vi "CI Server Build Package.vi"() -> ()   [LabVIEW 2016]
doc: "This VI is an example of a VI that can build a VIPM Package when the Build button is pushed or when called from the command line."
uses:
  <vilib>/SourceControl/sccapi/SCCAPI Refnum.ctl
  <userlib>/_OpenG.lib/file/file.llb/File Exists - Scalar__ogtk.vi
  <userlib>/_OpenG.lib/file/file.llb/Valid Path - Traditional__ogtk.vi
  <vilib>/AppBuilder/AB_API_Simple/Build (path).vi
  <vilib>/AppBuilder/AB_API_Simple/NI_App_Builder_API.lvlib
  LabVIEW Project API__icon_lib_labview_project_api Folder/LabVIEW Project API__icon_lib_labview_project_api.lvlib
  <vilib>/SourceControl/sccapi/NI_SCC.lvlib
panel:
  out "Build Number":u32
  out "Tests Pass":bool
  out "Unit Test Results":string
  in  "VI Package Build Spec path":path
  in  "button_build":bool
  out "Progress status":string
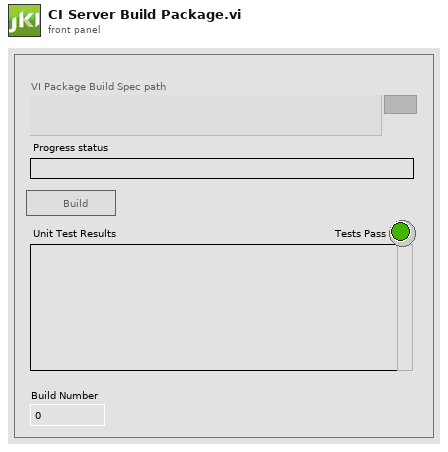
[diagram p1: front panel]
types:
  T1 = enum32{"invalid app kind", "Development System", "Run Time System", "Student Edition", "Embedded LabVIEW", "Evaluation", "Custom"}
  T2 = enum8{"Enabled", "Disabled", "Disabled and Grayed Out"}
  T3 = enum32{"Invalid", "Standard", "Closed", "Hidden", "Minimized", "Maximized"}
  T4 = typedef "NI_SCC.lvlib/SCCAPI Refnum.ctl" = refnum<k1>
  T5 = cluster{"Core":cluster{"Current VI Reference":refnum<vi>, "Close Panel on Exit?":bool}, "Paths":cluster{"Package Spec file path":path, "Unit Test Path":path}, "Building":bool, "RunningAsCmdLine":bool, "SCC Ref":T4, "Proj Ref":refnum<vi>, "Proj Item":refnum<vi>, "CmdLineArgs":cluster{"BuildNumber":u32, "Error Path":path, "Running Path":path, "Settings Path":path}}
  T6 = cluster{"BuildNumber":u32, "Error Path":path, "Running Path":path, "Settings Path":path}
  T7 = cluster{"Package Spec file path":path, "Unit Test Path":path}
  T8 = cluster{"Current VI Reference":refnum<vi>, "Close Panel on Exit?":bool}
  T9 = cluster{"Major":u16, "Minor":u16, "Fix":u16, "Build":u16}
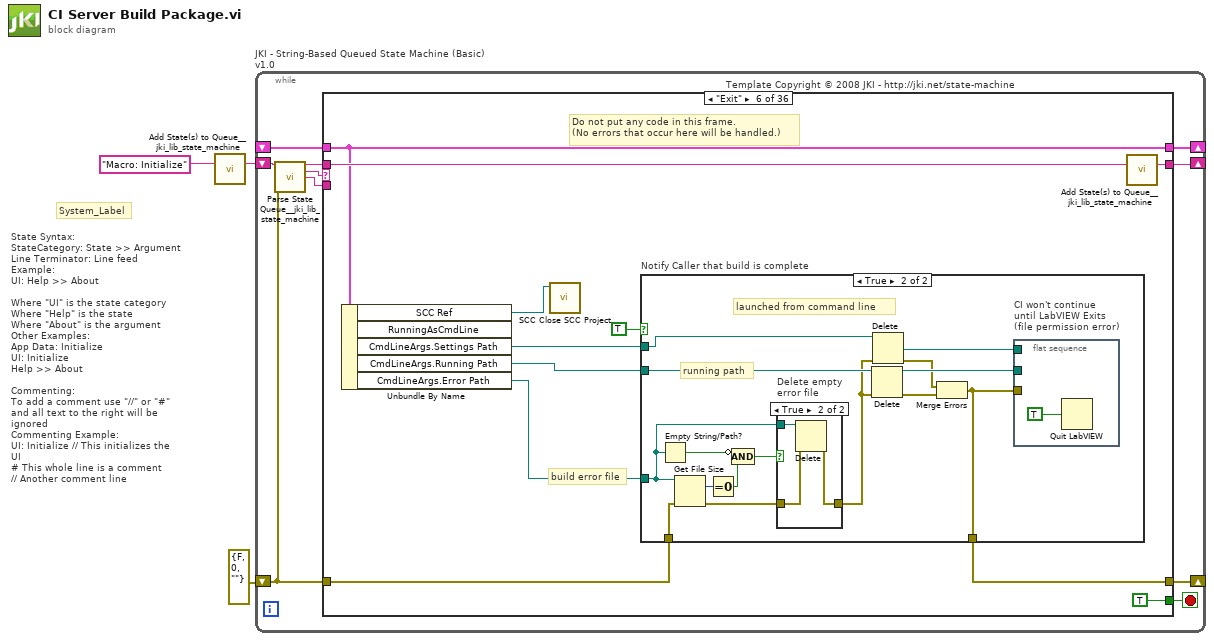
[diagram p0: block diagram]
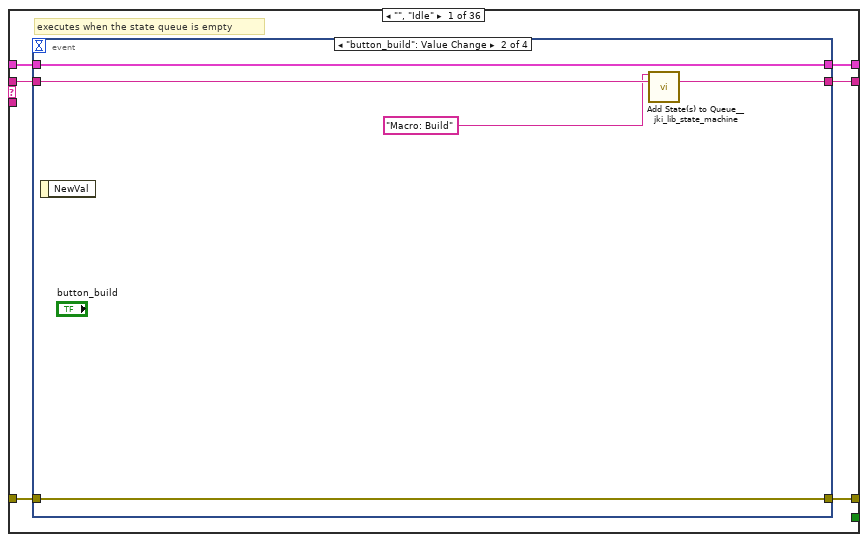
[diagram p2: hidden frame]
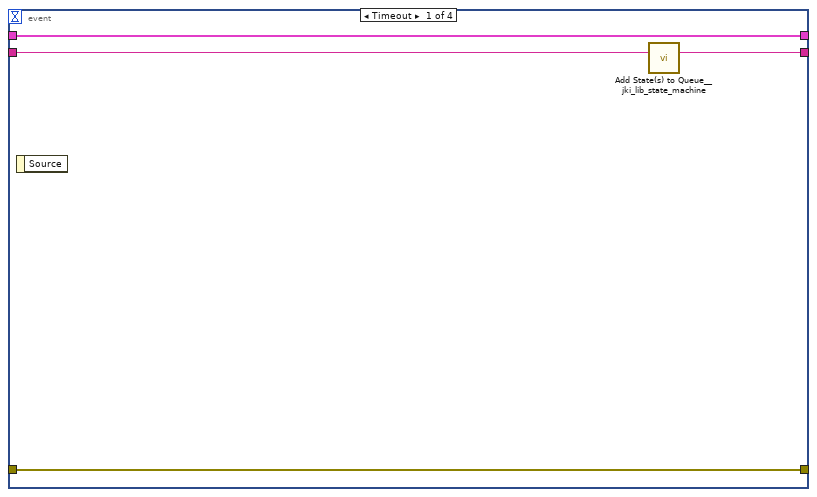
[diagram p3: hidden frame]
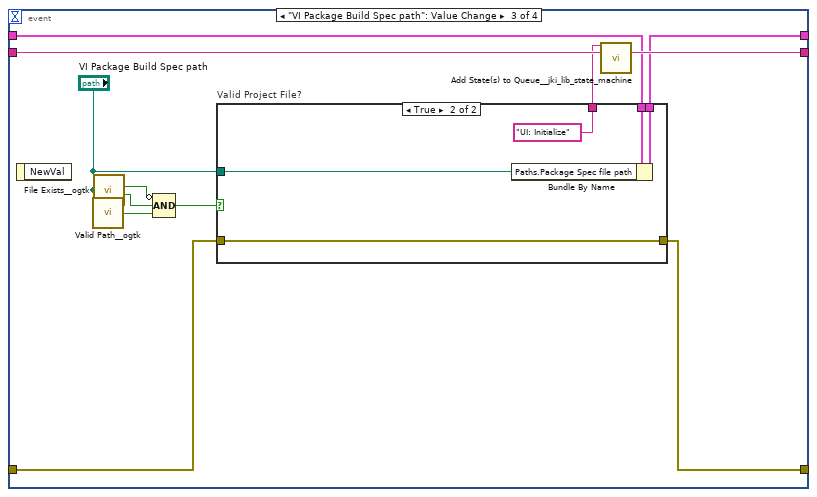
[diagram p4: hidden frame]
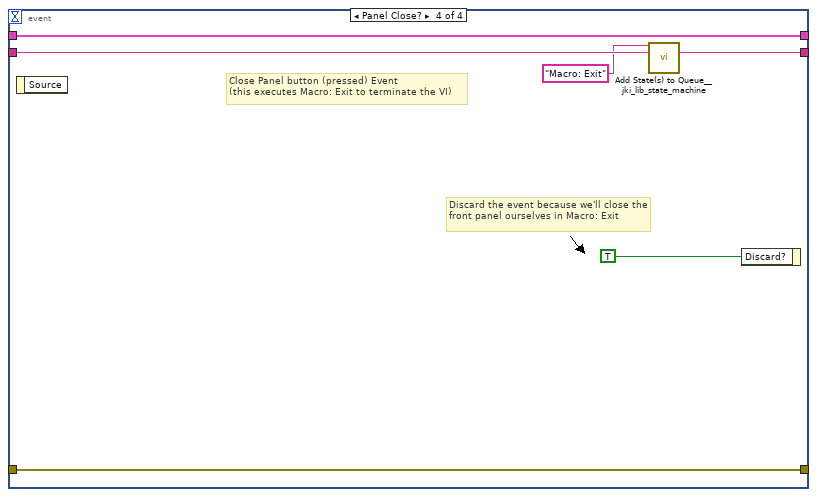
[diagram p6: hidden frame]
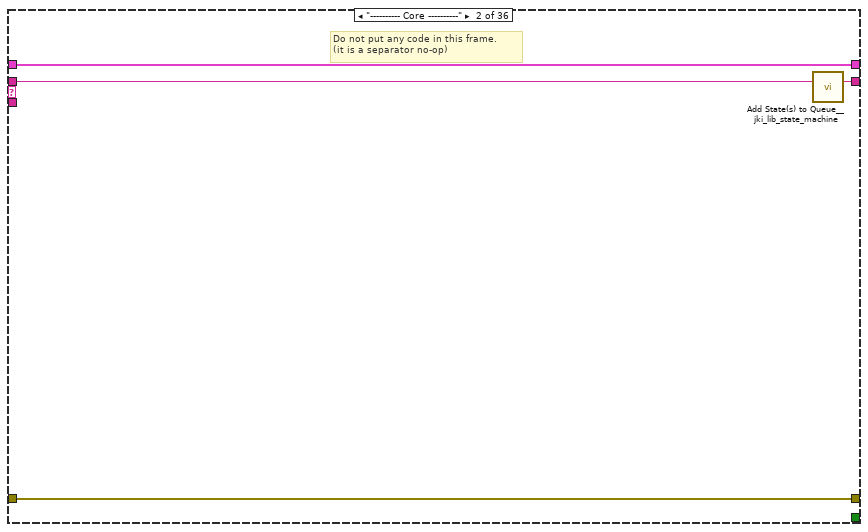
[diagram p7: hidden frame]
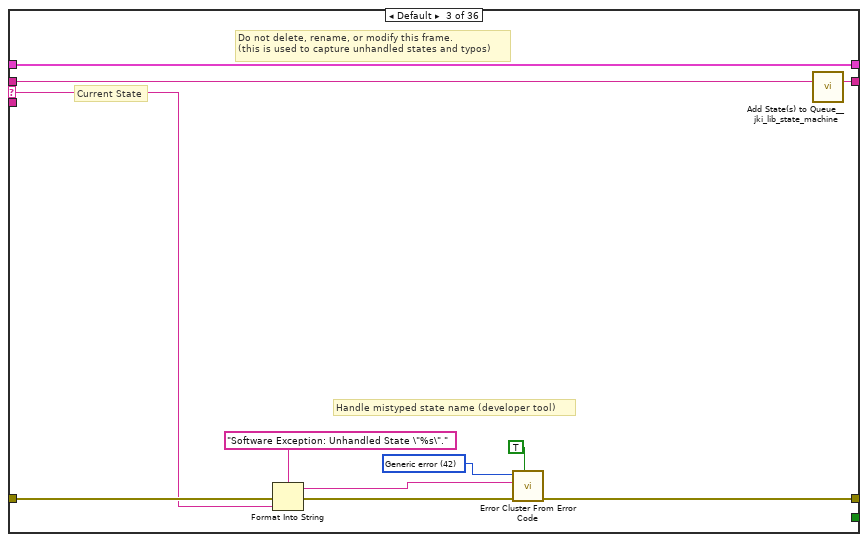
[diagram p8: hidden frame]
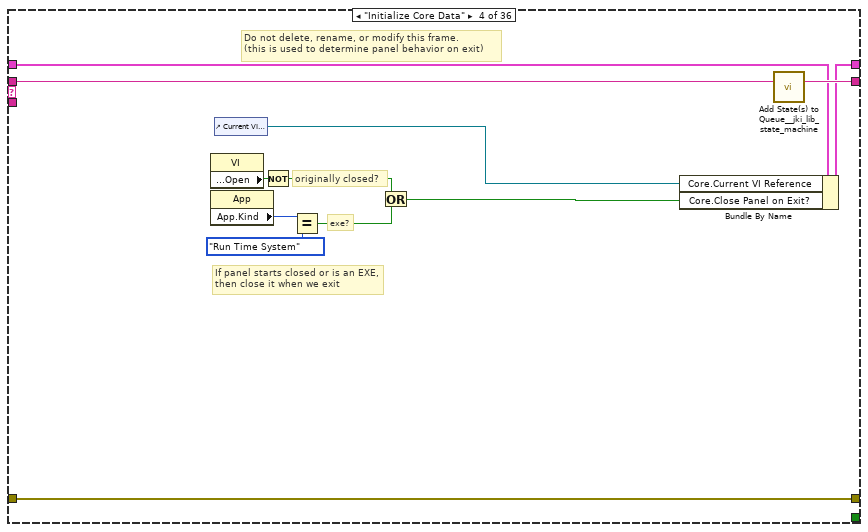
[diagram p9: hidden frame]
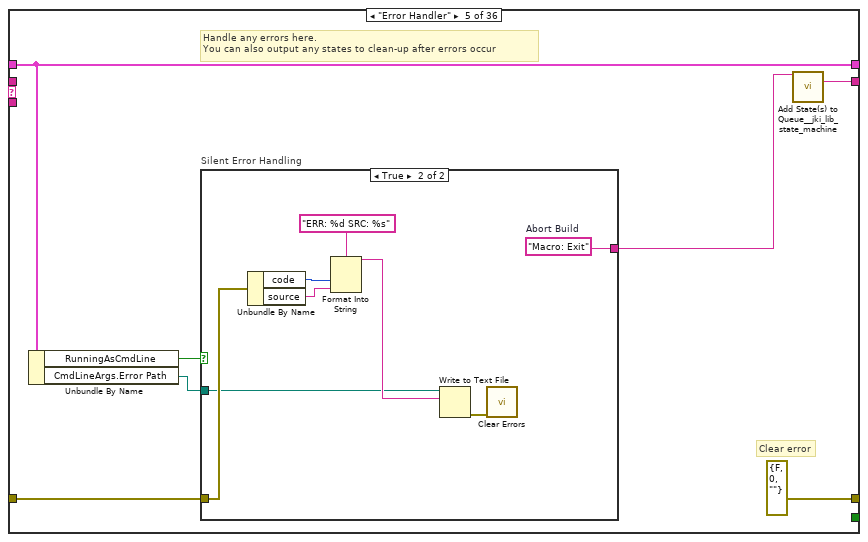
[diagram p10: hidden frame]
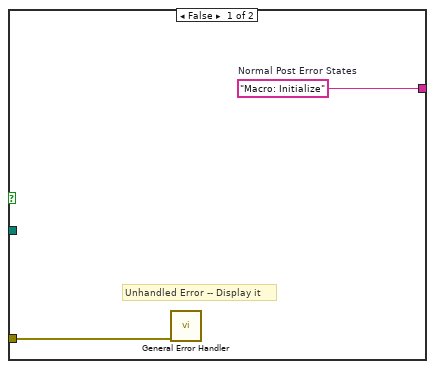
[diagram p11: hidden frame]
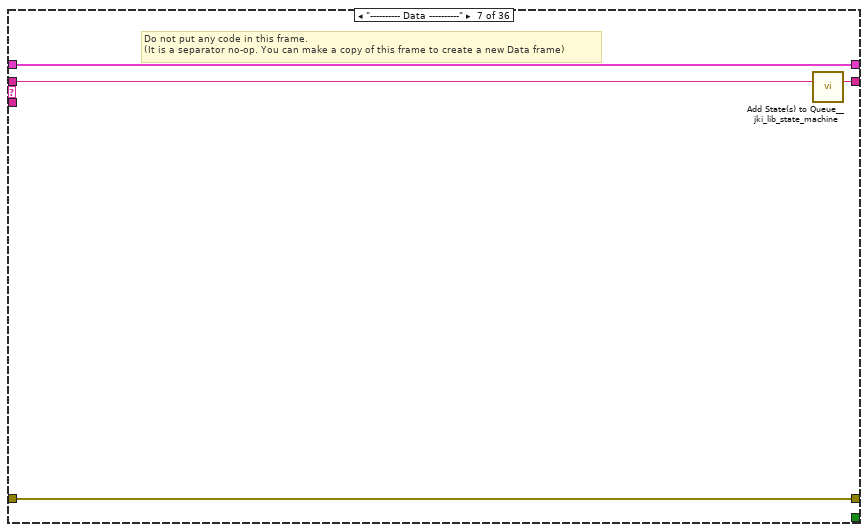
[diagram p14: hidden frame]
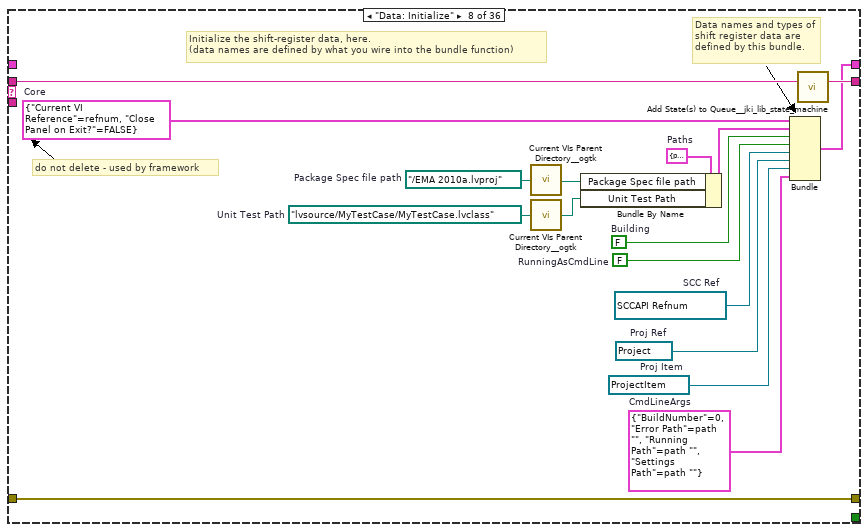
[diagram p15: hidden frame]
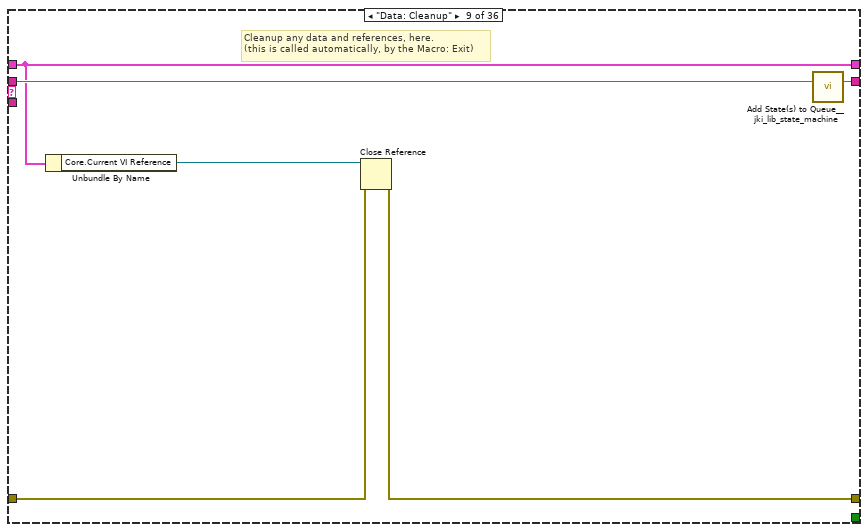
[diagram p16: hidden frame]
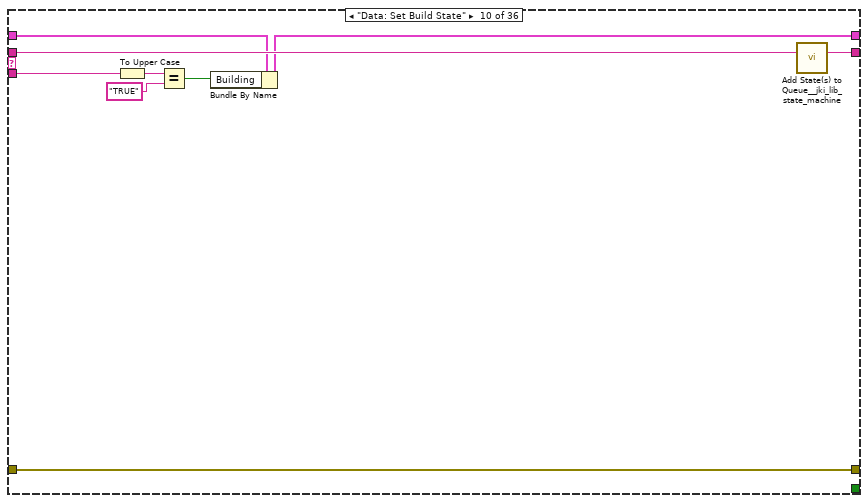
[diagram p17: hidden frame]
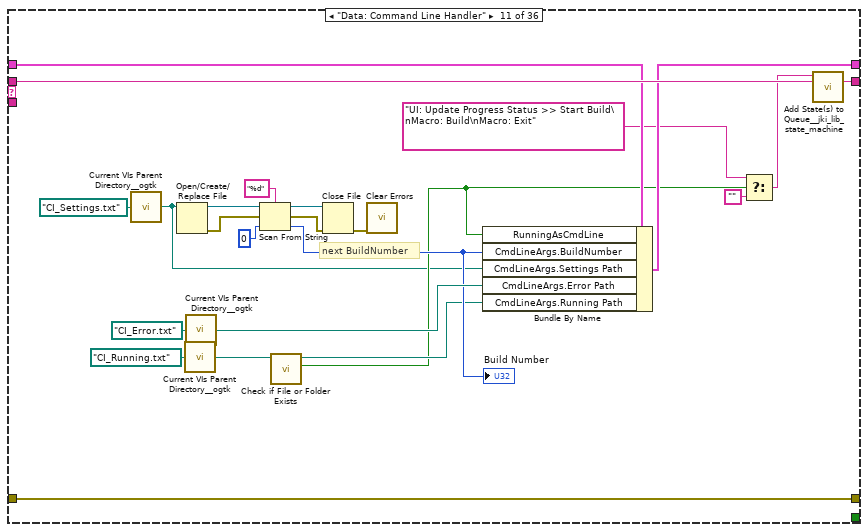
[diagram p18: hidden frame]
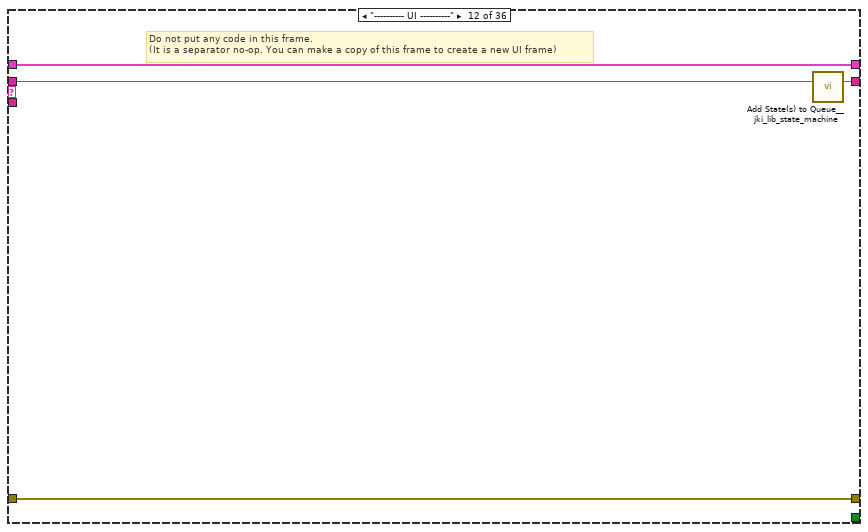
[diagram p19: hidden frame]
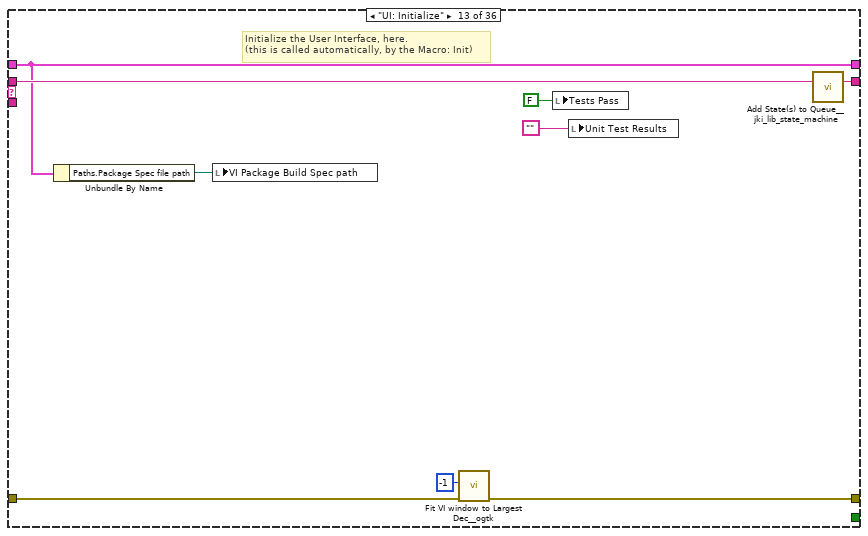
[diagram p20: hidden frame]
diagram:
  # "State Syntax:\nStateCategory: State >> Argument\nLine Terminator: Line feed\nExample:\nUI: Help >> About\n\nWhere \"UI\" is the state category\nWhere \"Help\" is the state\nWhere \"About\" is the argument\nOther Examples:\nApp Data: Initialize\nUI: Initialize\nHelp >> About\n\nCommenting:\nTo add a comment use \"//\" or \"#\" and all text to the right will be ignored\nCommenting Example:\nUI: Initialize // This initializes the UI\n# This whole line is a comment\n// Another comment line"
  # "System_Label"
  n1 = call <vilib>:"Add State(s) to Queue__jki_lib_state_machine.vi"("State(s) in (\"\")"="Macro: Initialize") -> ("States Out"=w1:string)  [unwired: 14 in]
  n2 = while "JKI - String-Based Queued State Machine (Basic) v1.0" {
    shift-right: [w6] -> _
    shift-left: _ -> [w5]
    shift-right: [w9] -> _
    shift-left: errorcluster {"status"=FALSE, "code"=0, "source"=""} ("error out") -> [w4]
    shift-right: [w8] -> _
    shift-left: w1 -> [w10]
    stop <- w7 stop-if-true
    # "Template Copyright © 2008 JKI - http://jki.net/state-machine"
    n3 = call <vilib>:"Parse State Queue__jki_lib_state_machine.vi"("State Queue"=w10, "Error In (no error)"=w4) -> ("Remaining States"=w12:string, "Current State"=w13:string, "Arguments"=w11:string)  [unwired: 11 in]
    n4 = case shown="\"Exit\"" w13 {
      selector: w13 -> [_ _ w58 _ _ _ _ _ _ _ _ _ _ _ _ _ _ _ _ _ _ _ _ _ _ _ _ _ _ _ _ _ _ _ _ _]
      tunnel: w12 -> [w19 w57 w62 w80 _ w108 w133 w150 w156 w165 w189 w193 w202 w207 w220 w238 w244 w255 w281 w286 w291 w296 w301 w311 w315 w318 w364 w375 w383 w394 w408 w418 w431 w440 w449 w470]
      tunnel: w11 -> [_ _ _ _ _ _ _ _ _ w159 _ _ _ _ w210 _ w239 w249 _ _ _ _ _ _ _ _ w359 _ _ _ _ _ _ _ _ w468]
      tunnel: w5 -> [w17 w54 w60 w71 w85 w103 w130 _ w151 w163 w187 w190 w200 w205 w218 w236 w242 w251 w278 w283 w288 w294 w298 w308 w312 w319 w362 w370 w381 w388 w405 w415 w420 w438 w447 w457]
      tunnel: [w16 w55 w64 w77 errorcluster {"status"=FALSE, "code"=0, "source"=""} ("error out") w104 w131 w140 w152 w162 w183 w191 w196 w204 w216 w235 w240 w252 w279 w284 w289 w293 w299 w309 w313 w316 w358 w365 w376 w391 w396 w410 w422 w433 w443 w450] -> w9
      tunnel: w4 -> [w15 w55 w63 w77 w83 w105 w131 w140 w153 w162 w183 w191 w199 w204 w217 w235 w241 w253 w279 w284 w289 w293 w299 w309 w313 w317 w361 w367 w377 w386 w401 w411 w423 w434 w442 w458]
      tunnel: [w18 w56 w61 w79 w87 w107 w132 w149 w155 w164 w188 w192 w201 w206 w219 w237 w243 w254 w280 w285 w290 w295 w300 w310 w314 w320 w363 w374 w382 w393 w407 w417 w430 w439 w448 w469] -> w8
      tunnel: [_ _ _ _ _ TRUE _ _ _ _ _ _ _ _ _ _ _ _ _ _ _ _ _ _ _ _ _ _ _ _ _ _ _ _ _ _] -> w7
      tunnel: [w14 w54 w60 w78 w85 w103 w130 w148 w151 w161 w186 w190 w200 w205 w218 w236 w242 w251 w278 w283 w288 w294 w298 w308 w312 w319 w362 w369 w380 w388 w404 w414 w419 w437 w446 w456] -> w6
      frame "", "Idle" {
        # "executes when the state queue is empty"
        n5 = event shown="[1] \"button_build\": Value Change" {
          selector: _ -> [_ _ _ _]
          dyn-events: _ -> [_ _ _ _]
          timeout: _ -> [_ _ _ _]
          tunnel: w19 -> [w23 w28 w40 w53]
          tunnel: [w22 w27 w39 w52] -> w18
          tunnel: w17 -> [w20 w24 w34 w50]
          tunnel: [w21 w25 w30 w51] -> w16
          tunnel: w15 -> [w21 w25 w31 w51]
          tunnel: [w20 w24 w33 w50] -> w14
          event Timeout {
            n6 = event-data() -> ()  [unwired: 1 in, 1 out]
            n7 = call <vilib>:"Add State(s) to Queue__jki_lib_state_machine.vi"("State(s) in (\"\")"=w23) -> ("States Out"=w22:string)  [unwired: 14 in]
          }
          event "button_build": Value Change {
            n8 = event-data() -> ()  [unwired: 1 in, 1 out]
            n9 = call <vilib>:"Add State(s) to Queue__jki_lib_state_machine.vi"("State(s) in Front (\"\")"="Macro: Build", "State(s) in (\"\")"=w28) -> ("States Out"=w27:string)  [unwired: 13 in]
          }
          event "VI Package Build Spec path": Value Change {
            n10 = event-data() -> ()  [unwired: 1 in, 1 out]
            n11 = call-poly <userlib>:"Valid Path__ogtk.vi"("path"="VI Package Build Spec path") -> ("valid"=w38:bool)
            n12 = call-poly <userlib>:"File Exists__ogtk.vi"("file path"="VI Package Build Spec path") -> ("is directory"=w36:bool, "exists"=w37:bool)  [unwired: 6 in]
            n13 = Compound Arithmetic op=AND(invert w36, w37, w38) -> (w35:bool)
            n14 = case "Valid Project File?" shown="True" w35 {
              tunnel: w31 -> [w42 w43]
              tunnel: "VI Package Build Spec path" -> [_ w45]
              tunnel: w34 -> [w41 w47]
              tunnel: [w41 w46] -> w33
              tunnel: [_ "UI: Initialize"] -> w32
              tunnel: [w42 w43] -> w30
              frame False {
              }
              frame True {
                n15 = Bundle By Name(cluster=w47, "Paths.Package Spec file path"=w45) -> (w46:T5)
              }
            }
            n16 = call <vilib>:"Add State(s) to Queue__jki_lib_state_machine.vi"("State(s) in Front (\"\")"=w32, "State(s) in (\"\")"=w40) -> ("States Out"=w39:string)  [unwired: 13 in]
          }
          event Panel Close? {
            # "Discard the event because we'll close the front panel ourselves in Macro: Exit"
            # "Close Panel button (pressed) Event\n(this executes Macro: Exit to terminate the VI)"
            n17 = event-data() -> ()  [unwired: 1 in, 1 out]
            n18 = call <vilib>:"Add State(s) to Queue__jki_lib_state_machine.vi"("State(s) in Front (\"\")"="Macro: Exit", "State(s) in (\"\")"=w53) -> ("States Out"=w52:string)  [unwired: 13 in]
            n19 = event-data("Discard?"=TRUE) -> ()  [unwired: 1 in, 1 out]
          }
        }
      }
      frame "---------- Core ----------" {
        # "Do not put any code in this frame.\n(it is a separator no-op)"
        n20 = call <vilib>:"Add State(s) to Queue__jki_lib_state_machine.vi"("State(s) in (\"\")"=w57) -> ("States Out"=w56:string)  [unwired: 14 in]
      }
      frame Default {
        w67 = 42 items=["No error", "Argument error", "Memory is full", "Out of zone", "End of file", "File already open", "Generic file I/O error", "File not found", "File permission error", "Disk is full", "Duplicate path", "Too many files open", "System feature not enabled", "Resource file not found", "Cannot add resource", "Resource not found", "Image not found", "Image memory error", "Pen does not exist", "Config type invalid", "Config token not found", "Config parse error", "Config memory error", "Bad external code format", "Bad external code offset", "External code not present", "Null window", "Destroy window error", "Null menu", "Print aborted", "Bad print record", "Print driver error", "Windows error during printing", "Memory error during printing", "Print dialog error", "Generic print error", "Invalid device refnum", "Device not found", "Device parameter error", "Device unit error", "Cannot open device", "Device call aborted", "Generic error", "Cancelled by user", "Object ID too low", "Object ID too high", "Object not in heap", "Unknown heap", "Unknown object (invalid DefProc)", "Unknown object (DefProc not in table)", "Message out of range", "Invalid (null) method", "Unknown message", "Manager call not supported", "Bad address", "Network operation in progress", "Network operation timed out", "Connection is busy", "Network attribute not supported", "Network error", "Address in use", "System out of memory", "Connection aborted", "Connection refused", "Not connected", "Already connected", "Connection closed", "Initialization error (interapplication manager)", "Bad occurrence", "Wait on unbound occurrence handler", "Occurrence queue overflow", "Datalog type conflict", "Unused", "Unrecognized type (interapplication manager)", "Memory corrupt", "Failed to make temporary DLL", "Old CIN version", "Drag socket not found", "Failed to load drop-object", "Failed to register OLE object", "Failed to release OLE object", "Format specifier type mismatch", "Unknown format specifier", "Too few format specifiers", "Too many format specifiers", "Scan failed", "Newer CIN version", "Error converting to variant", "Runtime menu error", "Password tampered", "Variant attribute not found", "Incompatible variant data type", "Event data is not available", "Event Store is not present", "Occurrence is not found", "Event Queue is not created", "Event info is not available", "Refnum passed is NULL", "Error retrieving Class GUID", "Error retrieving CoClass GUID", "Error retrieving TypeLib GUID.", "Bad built application magic bytes.", "Specific driver is different from the specific driver associated with the Logical Name.", "There is no session opened to the class driver.", "Max Error", "MAX - Error with config objects", "MAX - Error loading configuration", "MAX - Group not supported"]
        # "Current State"
        # "Do not delete, rename, or modify this frame.\n(this is used to capture unhandled states and typos)"
        # "Handle mistyped state name (developer tool)"
        n21 = Format Into String(format string="Software Exception: Unhandled State \"%s\"." ("message"), error in=w63, w58) -> (resulting string=w66:string, error out=w65:errorcluster)  [unwired: 1 in]
        n22 = call <vilib>:"Error Cluster From Error Code.vi"("show call chain? (False)"=TRUE, "error in (no error)"=w65, "error message (\"\")"=w66, "error code (0)"=w67) -> ("error out"=w64:errorcluster)  [unwired: 5 in]
        n23 = call <vilib>:"Add State(s) to Queue__jki_lib_state_machine.vi"("State(s) in (\"\")"=w62) -> ("States Out"=w61:string)  [unwired: 14 in]
      }
      frame "Initialize Core Data" {
        # "Do not delete, rename, or modify this frame.\n(this is used to determine panel behavior on exit)"
        # "originally closed?"
        # "exe?"
        # "If panel starts closed or is an EXE, then close it when we exit"
        n24 = property class="VI"() -> ("Front Panel.Open"=w76:bool)  [unwired: 2 in, 2 out]
        n25 = property class="App"() -> ("App.Kind"=w75:T1)  [unwired: 2 in, 2 out]
        n26 = control-ref of="Current VI Reference"() -> (w69:refnum<vi>)
        n27 = Not(x=w76) -> (.not. x?=w73:bool)
        n28 = Equal?(x=w75, y=T1."Run Time System" ("Application:Kind")) -> (x = y?=w72:bool)
        n29 = Or(x=w73, y=w72) -> (x .or. y?=w70:bool)
        n30 = Bundle By Name(cluster=w71, "Core.Current VI Reference"=w69, "Core.Close Panel on Exit?"=w70) -> (w78:T5)
        n31 = call <vilib>:"Add State(s) to Queue__jki_lib_state_machine.vi"("State(s) in (\"\")"=w80) -> ("States Out"=w79:string)  [unwired: 14 in]
      }
      frame "Error Handler" {
        # "Handle any errors here.\nYou can also output any states to clean-up after errors occur"
        # "Clear error"
        n32 = Unbundle By Name(w85) -> ("RunningAsCmdLine"=w84:bool, "CmdLineArgs.Error Path"=w81:path)
        n33 = case "Silent Error Handling" shown="True" w84 {
          tunnel: w83 -> [w89 w92]
          tunnel: [w88 w93] -> w82
          tunnel: w81 -> [_ w90]
          frame False {
            w88 = "Macro: Initialize"  # Normal Post Error States
            # "Unhandled Error -- Display it"
            n34 = call <vilib>:"General Error Handler.vi"("error in (no error)"=w89) -> ()  [unwired: 10 in, 5 out]
          }
          frame True {
            w93 = "Macro: Exit"  # Abort Build
            n35 = Unbundle By Name(w92) -> ("code"=w95:i32, "source"=w97:string)
            n36 = Format Into String(format string="ERR: %d SRC: %s", w95, w97) -> (resulting string=w94:string)  [unwired: 2 in, 1 out]
            n37 = Write to Text File(file (use dialog)=w90, text=w94) -> (error out=w91:errorcluster)  [unwired: 2 in, 2 out]
            n38 = call <vilib>:"Clear Errors.vi"("error in (no error)"=w91) -> ()  [unwired: 5 in, 2 out]
          }
        }
        n39 = call <vilib>:"Add State(s) to Queue__jki_lib_state_machine.vi"("State(s) in Front (\"\")"=w82) -> ("States Out"=w87:string)  [unwired: 14 in]
      }
      frame "Exit" {
        # "build error file"
        # "Do not put any code in this frame.\n(No errors that occur here will be handled.)"
        n40 = Unbundle By Name(w103) -> ("SCC Ref"=w99:T4, "CmdLineArgs.Settings Path"=w100:path, "CmdLineArgs.Running Path"=w102:path, "CmdLineArgs.Error Path"=w101:path)  [unwired: 1 out]
        n41 = call <vilib>:"SCC Close SCC Project.vi"("source control reference in"=w99) -> ()  [unwired: 9 in, 2 out]
        n42 = case "Notify Caller that build is complete" shown="True" TRUE {
          tunnel: w102 -> [_ w116]
          tunnel: w105 -> [w109 w122]
          tunnel: [w109 w110] -> w104
          tunnel: w101 -> [_ w120]
          tunnel: w100 -> [_ w115]
          frame False {
          }
          frame True {
            # "running path"
            # "launched from command line"
            n43 = Empty String/Path?(string/path=w120) -> (empty?=w119:bool)
            n44 = Get File Size(file=w120, error in=w122) -> (size (in bytes)=w123:i64, 0:w121:errorcluster)  [unwired: 1 out]
            n45 = Equal To 0?(x=w123) -> (x = 0?=w118:bool)
            n46 = Compound Arithmetic op=AND(invert w119, w118) -> (w117:bool)
            n47 = case "Delete empty\nerror file" shown="True" w117 {
              tunnel: w120 -> [_ w128]
              tunnel: w121 -> [w125 w127]
              tunnel: [w125 w126] -> w113
              frame False {
              }
              frame True {
                n48 = Delete(path (use dialog)=w128, error in=w127) -> (error out=w126:errorcluster)  [unwired: 3 in, 2 out]
              }
            }
            n49 = Delete(path (use dialog)=w116, error in=w113) -> (deleted path=w124:path, error out=w111:errorcluster)  [unwired: 3 in, 1 out]
            n50 = Delete(path (use dialog)=w115, error in=w113) -> (deleted path=w114:path, error out=w112:errorcluster)  [unwired: 3 in, 1 out]
            n51 = Merge Errors(w112, w111) -> (w110:errorcluster)
            n52 = flat-sequence "CI won't continue\nuntil LabVIEW Exits\n(file permission error)" {
              tunnel: w124 -> [_]
              tunnel: w114 -> [_]
              tunnel: w110 -> [_]
              frame #0 {
                n53 = Quit LabVIEW(quit? (T)=TRUE) -> ()
              }
            }
          }
        }
        n54 = call <vilib>:"Add State(s) to Queue__jki_lib_state_machine.vi"("State(s) in (\"\")"=w108) -> ("States Out"=w107:string)  [unwired: 14 in]
      }
      frame "---------- Data ----------" {
        # "Do not put any code in this frame.\n(It is a separator no-op. You can make a copy of this frame to create a new Data frame)"
        n55 = call <vilib>:"Add State(s) to Queue__jki_lib_state_machine.vi"("State(s) in (\"\")"=w133) -> ("States Out"=w132:string)  [unwired: 14 in]
      }
      frame "Data: Initialize" {
        w134 = refnum<vi> refnum  # Proj Item
        w135 = refnum<vi> refnum  # Proj Ref
        w136 = T4 refnum items=["SourceControl"]  # SCC Ref
        w137 = T6 {"BuildNumber"=0, "Error Path"=path "", "Running Path"=path "", "Settings Path"=path ""}  # CmdLineArgs
        w144 = path "lvsource/MyTestCase/MyTestCase.lvclass"  # Unit Test Path
        w145 = path "../EMA 2010a.lvproj"  # Package Spec file path
        w138 = FALSE  # RunningAsCmdLine
        w146 = T7 {"Package Spec file path"=path "", "Unit Test Path"=path ""}  # Paths
        w139 = FALSE  # Building
        w147 = T8 {"Current VI Reference"=refnum, "Close Panel on Exit?"=FALSE}  # Core
        # "do not delete - used by framework"
        # "Data names and types of shift register data are defined by this bundle."
        # "Initialize the shift-register data, here.\n(data names are defined by what you wire into the bundle function)"
        n56 = call <userlib>:"Current VIs Parent Directory__ogtk.vi"("Relative path (.)"=w145) -> ("Parent Directory (+ Relative)"=w142:path)  [unwired: 4 in]
        n57 = call <userlib>:"Current VIs Parent Directory__ogtk.vi"("Relative path (.)"=w144) -> ("Parent Directory (+ Relative)"=w141:path)  [unwired: 4 in]
        n58 = Bundle By Name(cluster=w146, "Package Spec file path"=w142, "Unit Test Path"=w141) -> (w143:T7)
        n59 = Bundle("Core"=w147, "Paths"=w143, "Building"=w139, "RunningAsCmdLine"=w138, "SCC Ref"=w136, "Proj Ref"=w135, "Proj Item"=w134, "CmdLineArgs"=w137) -> (w148:T5)  [unwired: 1 in]
        n60 = call <vilib>:"Add State(s) to Queue__jki_lib_state_machine.vi"("State(s) in (\"\")"=w150) -> ("States Out"=w149:string)  [unwired: 14 in]
      }
      frame "Data: Cleanup" {
        # "Cleanup any data and references, here.\n(this is called automatically, by the Macro: Exit)"
        n61 = Unbundle By Name(w151) -> ("Core.Current VI Reference"=w154:refnum<vi>)
        n62 = Close Reference(reference=w154, error in (no error)=w153) -> (error out=w152:errorcluster)
        n63 = call <vilib>:"Add State(s) to Queue__jki_lib_state_machine.vi"("State(s) in (\"\")"=w156) -> ("States Out"=w155:string)  [unwired: 14 in]
      }
      frame "Data: Set Build State" {
        n64 = To Upper Case(1:w159) -> (0:w160:string)
        n65 = Equal?(x=w160, y="TRUE") -> (x = y?=w157:bool)
        n66 = Bundle By Name(cluster=w163, "Building"=w157) -> (w161:T5)
        n67 = call <vilib>:"Add State(s) to Queue__jki_lib_state_machine.vi"("State(s) in (\"\")"=w165) -> ("States Out"=w164:string)  [unwired: 14 in]
      }
      frame "Data: Command Line Handler" {
        # "next BuildNumber"
        n68 = call <userlib>:"Current VIs Parent Directory__ogtk.vi"("Relative path (.)"=path "CI_Settings.txt") -> ("Parent Directory (+ Relative)"=w170:path)  [unwired: 4 in]
        n69 = Open/Create/Replace File(file path (use dialog)=w170) -> (refnum out=w177:refnum<file>, error out=w168:errorcluster)  [unwired: 5 in, 1 out]
        n70 = call <userlib>:"Current VIs Parent Directory__ogtk.vi"("Relative path (.)"=path "CI_Running.txt") -> ("Parent Directory (+ Relative)"=w173:path)  [unwired: 4 in]
        n71 = call <userlib>:"Current VIs Parent Directory__ogtk.vi"("Relative path (.)"=path "CI_Error.txt") -> ("Parent Directory (+ Relative)"=w179:path)  [unwired: 4 in]
        n72 = Scan From String("%d" ("format string"), w177, w168, default 1=u32 0 ("default value 1")) -> (w169:refnum<file>, w167:errorcluster, output 1=w175:u32)
        "Build Number" <- w175
        n73 = call <vilib>:"Check if File or Folder Exists.vi"("path"=w173) -> ("file or folder exists?"=w171:bool, "dup path"=w172:path)  [unwired: 8 in, 1 out]
        n74 = Close File(refnum=w169, error in=w167) -> (error out=w166:errorcluster)  [unwired: 1 out]
        n75 = call <vilib>:"Clear Errors.vi"("error in (no error)"=w166) -> ()  [unwired: 5 in, 2 out]
        n76 = Bundle By Name(cluster=w187, "RunningAsCmdLine"=w171, "CmdLineArgs.BuildNumber"=w175, "CmdLineArgs.Settings Path"=w170, "CmdLineArgs.Error Path"=w179, "CmdLineArgs.Running Path"=w172) -> (w186:T5)
        n77 = Select(t="UI: Update Progress Status >> Start Build\nMacro: Build\nMacro: Exit", s=w171, f="") -> (s? t:f=w184:string)
        n78 = call <vilib>:"Add State(s) to Queue__jki_lib_state_machine.vi"("State(s) in Front (\"\")"=w184, "State(s) in (\"\")"=w189) -> ("States Out"=w188:string)  [unwired: 13 in]
      }
      frame "---------- UI ----------" {
        # "Do not put any code in this frame.\n(It is a separator no-op. You can make a copy of this frame to create a new UI frame)"
        n79 = call <vilib>:"Add State(s) to Queue__jki_lib_state_machine.vi"("State(s) in (\"\")"=w193) -> ("States Out"=w192:string)  [unwired: 14 in]
      }
      frame "UI: Initialize" {
        # "Initialize the User Interface, here.\n(this is called automatically, by the Macro: Init)"
        n80 = Unbundle By Name(w200) -> ("Paths.Package Spec file path"=w195:path)
        n81 = local write "VI Package Build Spec path"(w195) -> ()
        n82 = call <userlib>:"Fit VI window to Largest Dec__ogtk.vi"("error in (no error)"=w199, "border spacing (2 px)"=-1) -> ("error out"=w196:errorcluster)  [unwired: 4 in, 1 out]
        n83 = local write "Tests Pass"(FALSE ("Unit Tests Pass")) -> ()
        n84 = local write "Unit Test Results"("") -> ()
        n85 = call <vilib>:"Add State(s) to Queue__jki_lib_state_machine.vi"("State(s) in (\"\")"=w202) -> ("States Out"=w201:string)  [unwired: 14 in]
      }
      frame "UI: Reset Progress Status" {
        n86 = call <vilib>:"Add State(s) to Queue__jki_lib_state_machine.vi"("State(s) in Front (\"\")"="UI: Update Progress Status >> Idle" ("State(s) in Front (\"\")"), "State(s) in (\"\")"=w207) -> ("States Out"=w206:string)  [unwired: 13 in]
      }
      frame "UI: Update Progress Status" {
        # "A delay allows this command to\nbe captured by the bash script\nstatus display."
        n87 = Unbundle By Name(w218) -> ("CmdLineArgs.Running Path"=w213:path)
        n88 = Empty String/Path?(string/path=w213) -> (empty?=w212:bool)
        n89 = Wait (ms)(milliseconds to wait=u32 200) -> ()  [unwired: 1 out]
        n90 = case shown="False" w212 {
          tunnel: [w223 w225] -> w215
          tunnel: [w222 FALSE ("file or folder exists?")] -> w214
          tunnel: w213 -> [w221 w225]
          frame False {
            n91 = call <vilib>:"Check if File or Folder Exists.vi"("path"=w221) -> ("file or folder exists?"=w222:bool, "dup path"=w223:path)  [unwired: 8 in, 1 out]
          }
          frame True {
          }
        }
        n92 = Concatenate Strings(w210, "\r\n") -> (w209:string)
        n93 = case shown="True" w214 {
          tunnel: w215 -> [_ w230]
          tunnel: w209 -> [_ w229]
          tunnel: w217 -> [w226 w228]
          tunnel: [w226 w227] -> w216
          frame False {
          }
          frame True {
            n94 = Write to Text File(file (use dialog)=w230, text=w229, error in=w228) -> (error out=w227:errorcluster)  [unwired: 1 in, 2 out]
          }
        }
        n95 = call <vilib>:"Add State(s) to Queue__jki_lib_state_machine.vi"("State(s) in (\"\")"=w220) -> ("States Out"=w219:string)  [unwired: 14 in]
        "Progress status" <- w210
      }
      frame "UI: Update Interlock" {
        n96 = Unbundle By Name(w236) -> ("Building"=w232:bool)
        n97 = Select(t=T2."Disabled and Grayed Out" ("Disabled"), s=w232, f=T2."Enabled" ("Disabled")) -> (s? t:f=w231:T2)
        n98 = property on="button_build" class="Bool"("DisabledEnum"=w231) -> ()  [unwired: 2 in, 2 out]
        n99 = property on="VI Package Build Spec path" class="Path"("DisabledEnum"=w231) -> ()  [unwired: 2 in, 2 out]
        n100 = call <vilib>:"Add State(s) to Queue__jki_lib_state_machine.vi"("State(s) in (\"\")"=w238) -> ("States Out"=w237:string)  [unwired: 14 in]
      }
      frame "UI: Cursor Set" {
        # "Argument"
        # "Set and Unset Cursor Busy.\n(Usage: \"UI: Cursor Set >> Busy|Idle\")"
        n101 = case shown="\"Idle\", Default" w239 {
          tunnel: w241 -> [w246 w248]
          tunnel: [w245 w247] -> w240
          frame "Idle", Default {
            n102 = call <vilib>:"Unset Busy.vi"("error in (no error)"=w246) -> ("error out"=w245:errorcluster)  [unwired: 10 in]
          }
          frame "Busy" {
            n103 = call <vilib>:"Set Busy.vi"("error in (no error)"=w248) -> ("error out"=w247:errorcluster)  [unwired: 9 in, 1 out]
          }
        }
        n104 = call <vilib>:"Add State(s) to Queue__jki_lib_state_machine.vi"("State(s) in (\"\")"=w244) -> ("States Out"=w243:string)  [unwired: 14 in]
      }
      frame "UI: Front Panel State" {
        # "Argument"
        # "Set Front Panel Open or Closed\n(Usage: \"UI: Front Panel State >> Open|Close\")"
        n105 = Unbundle By Name(w251) -> ("Core.Current VI Reference"=w250:refnum<vi>)
        n106 = case shown="\"Close\"" w249 {
          tunnel: w253 -> [w259 w272]
          tunnel: [w261 w273] -> w252
          tunnel: w250 -> [w260 w270]
          frame "Open", Default {
            n107 = property class="VI"(reference=w260, error in=w259) -> (reference out=w257:refnum<vi>, error out=w258:errorcluster, "Front Panel.Open"=w256:bool)
            n108 = case shown="True" w256 {
              tunnel: [w264 w267] -> w261
              tunnel: w258 -> [w263 w267]
              tunnel: w257 -> [w262 _]
              frame False {
                n109 = invoke class="VI" method="FP.Open"(reference=w262, error in=w263, "Activate"=TRUE, "State"=T3."Standard") -> (error out=w264:errorcluster)  [unwired: 1 in, 4 out]
              }
              frame True {
              }
            }
          }
          frame "Close" {
            n110 = property class="VI"(reference=w270, error in=w272) -> (reference out=w269:refnum<vi>, error out=w271:errorcluster, "Front Panel.Open"=w268:bool)
            n111 = case shown="True" w268 {
              tunnel: [w274 w277] -> w273
              tunnel: w271 -> [w274 w276]
              tunnel: w269 -> [_ w275]
              frame False {
              }
              frame True {
                n112 = invoke class="VI" method="FP.Close"(reference=w275, error in=w276) -> (error out=w277:errorcluster)  [unwired: 1 in, 2 out]
              }
            }
          }
        }
        n113 = call <vilib>:"Add State(s) to Queue__jki_lib_state_machine.vi"("State(s) in (\"\")"=w255) -> ("States Out"=w254:string)  [unwired: 14 in]
      }
      frame "---------- Macro ----------" {
        # "Do not put any code in this frame.\n(It is a separator no-op. You can make a copy of this frame to create a new Macro frame)"
        n114 = call <vilib>:"Add State(s) to Queue__jki_lib_state_machine.vi"("State(s) in (\"\")"=w281) -> ("States Out"=w280:string)  [unwired: 14 in]
      }
      frame "Macro: Initialize" {
        # "Initialization Macro\n(This is called once, when the VI starts)"
        n115 = call <vilib>:"Add State(s) to Queue__jki_lib_state_machine.vi"("State(s) in Front (\"\")"="Data: Initialize\nInitialize Core Data\nUI: Initialize\nUI: Update Interlock\nUI: Reset Progress Status\nUI: Front Panel State >> Open\nData: Command Line Handler", "State(s) in (\"\")"=w286) -> ("States Out"=w285:string)  [unwired: 13 in]
      }
      frame "Macro: Start Build" {
        n116 = call <vilib>:"Add State(s) to Queue__jki_lib_state_machine.vi"("State(s) in Front (\"\")"="Data: Set Build State >> True\nUI: Update Interlock", "State(s) in (\"\")"=w291) -> ("States Out"=w290:string)  [unwired: 13 in]
      }
      frame "Macro: Build" {
        n117 = call <vilib>:"Add State(s) to Queue__jki_lib_state_machine.vi"("State(s) in Front (\"\")"="Macro: Start Build\nUI: Update Progress Status >> Load Project File\nProject: Check out\nProject: Load\nUI: Update Progress Status >> Running Unit Tests ...\nProject: Run Unit Tests\n//\nUI: Update Progress Status >> Process EMA2010 DC Daemon\nUI: Update Progress Status >> Update Build Number\nProject: Get Project Item >> EMA2010 DC Daemon\nProject: Enable Logfile\nProject: Set Build Number\nUI: Update Progress Status >> Building DC Daemon\nProject: Build >> EMA2010 DC Daemon\n//\nUI: Update Progress Status >> Process Eye Movement Analyser\nUI: Update Progress Status >> Update Build Number\nProject: Get Project Item >> Eye Movement Analyser\nProject: Enable Logfile\nProject: Set Build Number\nUI: Update Progress Status >> Building Eye Movement Analyser\nProject: Build >> Eye Movement Analyser\n//\nUI: Update Progress Status >> Process Installer\nUI: Update Progress Status >> Update Build Number\nProject: Get Project Item >> EMA 2010 installer\nProject: Set Installer Build Dir\nUI: Update Progress Status >> Building Installer\nProject: Build >> EMA 2010 installer\n//\nUI: Update Progress Status >> Close Project File\nProject: Close\nProject: Undo Check out\nUI: Update Progress Status >> Done\nMacro: End Build\n", "State(s) in (\"\")"=w296) -> ("States Out"=w295:string)  [unwired: 13 in]
      }
      frame "Macro: End Build" {
        n118 = call <vilib>:"Add State(s) to Queue__jki_lib_state_machine.vi"("State(s) in Front (\"\")"="Data: Set Build State >> False\nUI: Update Interlock", "State(s) in (\"\")"=w301) -> ("States Out"=w300:string)  [unwired: 13 in]
      }
      frame "Macro: Exit" {
        # "Exit Macro\n(This is called once, when the VI exits)"
        n119 = Unbundle By Name(w308) -> ("Core.Close Panel on Exit?"=w307:bool)
        n120 = Select(t="UI: Front Panel State >> Close", s=w307, f="") -> (s? t:f=w304:string)
        n121 = call <vilib>:"Add State(s) to Queue__jki_lib_state_machine.vi"("State(s) in (\"\")"=w304, "State(s) at Back (\"\")"="Data: Cleanup\nExit") -> ("States Out"=w302:string)  [unwired: 13 in]
        n122 = call <vilib>:"Add State(s) to Queue__jki_lib_state_machine.vi"("State(s) in Front (\"\")"=w302, "State(s) in (\"\")"=w311) -> ("States Out"=w310:string)  [unwired: 13 in]
      }
      frame "---------- Project ----------" {
        n123 = call <vilib>:"Add State(s) to Queue__jki_lib_state_machine.vi"("State(s) in (\"\")"=w315) -> ("States Out"=w314:string)  [unwired: 14 in]
      }
      frame "Project: Run Unit Tests" {
        n124 = disable-structure shown="Enabled" {
          disable-tunnel: [w342 w356] -> w320
          disable-tunnel: w319 -> [w341 _]
          disable-tunnel: w318 -> [w339 w355]
          disable-tunnel: w317 -> [w332 w357]
          disable-tunnel: [w327 w357] -> w316
          frame Disabled {
            # "Tests pass"
            n125 = Unbundle By Name(w341) -> ("RunningAsCmdLine"=w340:bool, "Paths.Unit Test Path"=w330:path)
            n126 = property on="Tests Pass" class="Bool (strict)"(error in=w332, "Value"=FALSE ("Unit Tests Pass")) -> (error out=w329:errorcluster)  [unwired: 1 in, 1 out]
            n127 = call <userlib>:"Current VIs Parent Directory__ogtk.vi"("Relative path (.)"=path "Support VIs/Run Project Unit Tests Dynamically.vi" ("VI Path")) -> ("Parent Directory (+ Relative)"=w325:path)  [unwired: 4 in]
            n128 = Open VI Reference(type specifier VI Refnum (for type only)=refnum<vi> refnum, vi path=w325, error in (no error)=w329) -> (vi reference=w336:refnum<vi>, error out=w335:errorcluster)  [unwired: 3 in]
            n129 = call-by-ref "?"(reference=w336, error in=w335, "error in"=w335, "TestSuite"=w330) -> (reference out=w334:refnum<vi>, error out=w333:errorcluster, 0:"error out"=w328:errorcluster, "test details"=w322:string, "successful?"=w323:bool)  [unwired: 7 in]
            "Tests Pass" <- w323
            "Unit Test Results" <- w322
            n130 = Close Reference(reference=w334, error in (no error)=w333) -> (error out=w326:errorcluster)
            n131 = case "Abort Build (Test Failure)" shown="False" w323 {
              tunnel: w340 -> [w347 _]
              tunnel: [w352 w354] -> w338
              tunnel: w339 -> [_ w354]
              tunnel: w322 -> [w350 _]
              tunnel: [w344 _] -> w321
              frame False {
                w343 = 42 items=["No error", "Argument error", "Memory is full", "Out of zone", "End of file", "File already open", "Generic file I/O error", "File not found", "File permission error", "Disk is full", "Duplicate path", "Too many files open", "System feature not enabled", "Resource file not found", "Cannot add resource", "Resource not found", "Image not found", "Image memory error", "Pen does not exist", "Config type invalid", "Config token not found", "Config parse error", "Config memory error", "Bad external code format", "Bad external code offset", "External code not present", "Null window", "Destroy window error", "Null menu", "Print aborted", "Bad print record", "Print driver error", "Windows error during printing", "Memory error during printing", "Print dialog error", "Generic print error", "Invalid device refnum", "Device not found", "Device parameter error", "Device unit error", "Cannot open device", "Device call aborted", "Generic error", "Cancelled by user", "Object ID too low", "Object ID too high", "Object not in heap", "Unknown heap", "Unknown object (invalid DefProc)", "Unknown object (DefProc not in table)", "Message out of range", "Invalid (null) method", "Unknown message", "Manager call not supported", "Bad address", "Network operation in progress", "Network operation timed out", "Connection is busy", "Network attribute not supported", "Network error", "Address in use", "System out of memory", "Connection aborted", "Connection refused", "Not connected", "Already connected", "Connection closed", "Initialization error (interapplication manager)", "Bad occurrence", "Wait on unbound occurrence handler", "Occurrence queue overflow", "Datalog type conflict", "Unused", "Unrecognized type (interapplication manager)", "Memory corrupt", "Failed to make temporary DLL", "Old CIN version", "Drag socket not found", "Failed to load drop-object", "Failed to register OLE object", "Failed to release OLE object", "Format specifier type mismatch", "Unknown format specifier", "Too few format specifiers", "Too many format specifiers", "Scan failed", "Newer CIN version", "Error converting to variant", "Runtime menu error", "Password tampered", "Variant attribute not found", "Incompatible variant data type", "Event data is not available", "Event Store is not present", "Occurrence is not found", "Event Queue is not created", "Event info is not available", "Refnum passed is NULL", "Error retrieving Class GUID", "Error retrieving CoClass GUID", "Error retrieving TypeLib GUID.", "Bad built application magic bytes.", "Specific driver is different from the specific driver associated with the Logical Name.", "There is no session opened to the class driver.", "Max Error", "MAX - Error with config objects", "MAX - Error loading configuration", "MAX - Group not supported"]
                n132 = Format Into String(format string="Unit test failures: %s", w350) -> (resulting string=w348:string)  [unwired: 2 in, 1 out]
                n133 = call <vilib>:"Error Cluster From Error Code.vi"("error message (\"\")"=w348, "error code (0)"=w343) -> ("error out"=w346:errorcluster)  [unwired: 7 in]
                n134 = Select(t=w346, s=w347, f=errorcluster {"status"=FALSE, "code"=0, "source"=""}) -> (s? t:f=w344:errorcluster)
                n135 = Select(t="Macro: Exit" ("Text.Text"), s=w347, f="UI: Update Progress Status >> Aborted: Unit Test Failure\nMacro: End Build" ("Text.Text")) -> (s? t:f=w352:string)
              }
              frame True {
              }
            }
            n136 = call <vilib>:"Add State(s) to Queue__jki_lib_state_machine.vi"("State(s) in (\"\")"=w338) -> ("States Out"=w342:string)  [unwired: 14 in]
            n137 = Merge Errors(w326, w328, w321) -> (w327:errorcluster)
          }
          frame Enabled {
            n138 = call <vilib>:"Add State(s) to Queue__jki_lib_state_machine.vi"("State(s) in (\"\")"=w355) -> ("States Out"=w356:string)  [unwired: 14 in]
          }
        }
      }
      frame "Project: Build" {
        n139 = Unbundle By Name(w362) -> ("Paths.Package Spec file path"=w360:path)  [unwired: 2 out]
        n140 = call-poly <vilib>:"Build.vi"("error in (no error)"=w361, "Name of build specification (if empty: build all)"=w359, "Path to project"=w360) -> ("error out"=w358:errorcluster)  [unwired: 7 in, 1 out]
        n141 = call <vilib>:"Add State(s) to Queue__jki_lib_state_machine.vi"("State(s) in (\"\")"=w364) -> ("States Out"=w363:string)  [unwired: 14 in]
      }
      frame "Project: Check out" {
        n142 = Unbundle By Name(w370) -> ("Paths.Package Spec file path"=w372:path)
        n143 = Build Array(w372) -> (w371:path[])
        n144 = call <vilib>:"SCC Open SCC Project.vi"("error in (no error)"=w367) -> ("error out"=w366:errorcluster, "source control reference out"=w373:T4)  [unwired: 8 in, 1 out]
        n145 = call <vilib>:"SCC Check Out.vi"("error in (no error)"=w366, "files"=w371, "source control reference in"=w373) -> ("error out"=w365:errorcluster, "source control reference out"=w368:T4)  [unwired: 5 in, 2 out]
        n146 = Bundle By Name(cluster=w370, "SCC Ref"=w368) -> (w369:T5)
        n147 = call <vilib>:"Add State(s) to Queue__jki_lib_state_machine.vi"("State(s) in (\"\")"=w375) -> ("States Out"=w374:string)  [unwired: 14 in]
      }
      frame "Project: Load" {
        n148 = Unbundle By Name(w381) -> ("Paths.Package Spec file path"=w379:path)
        n149 = call "Constructor__icon_lib_labview_project_api.vi"("error in (no error)"=w377, "Project Path"=w379) -> ("error out"=w376:errorcluster, "Project Reference"=w378:refnum<vi>)  [unwired: 8 in]
        n150 = Bundle By Name(cluster=w381, "Proj Ref"=w378) -> (w380:T5)
        n151 = call <vilib>:"Add State(s) to Queue__jki_lib_state_machine.vi"("State(s) in (\"\")"=w383) -> ("States Out"=w382:string)  [unwired: 14 in]
      }
      frame "Project: Close" {
        n152 = Unbundle By Name(w388) -> ("Proj Ref"=w392:refnum<vi>, "Proj Item"=w387:refnum<vi>)
        n153 = Close Reference(reference=w387, error in (no error)=w386) -> (error out=w385:errorcluster)
        n154 = call <vilib>:"Clear Errors.vi"("error in (no error)"=w385) -> ("error out"=w384:errorcluster)  [unwired: 5 in, 1 out]
        n155 = call "Destructor__icon_lib_labview_project_api.vi"("Close Project (F)"=TRUE, "error in (no error)"=w384, "Save Project (F)"=TRUE, "Project Reference"=w392) -> ("error out"=w391:errorcluster)  [unwired: 7 in]
        n156 = call <vilib>:"Add State(s) to Queue__jki_lib_state_machine.vi"("State(s) in (\"\")"=w394) -> ("States Out"=w393:string)  [unwired: 14 in]
      }
      frame "Project: Check in" {
        n157 = Unbundle By Name(w405) -> ("SCC Ref"=w403:T4, "Paths.Package Spec file path"=w406:path, "CmdLineArgs.BuildNumber"=w400:u32)
        n158 = Build Array(w406) -> (w402:path[])
        n159 = Number To Decimal String(number=w400) -> (decimal integer string=w399:string)  [unwired: 1 in]
        n160 = Concatenate Strings("Updated Project to Build Number ", w399) -> (w397:string)
        n161 = call <vilib>:"SCC Check In.vi"("error in (no error)"=w401, "comment"=w397, "files"=w402, "source control reference in"=w403) -> ("error out"=w396:errorcluster, "source control reference out"=w395:T4)  [unwired: 4 in, 2 out]
        n162 = Bundle By Name(cluster=w405, "SCC Ref"=w395) -> (w404:T5)
        n163 = call <vilib>:"Add State(s) to Queue__jki_lib_state_machine.vi"("State(s) in (\"\")"=w408) -> ("States Out"=w407:string)  [unwired: 14 in]
      }
      frame "Project: Undo Check out" {
        n164 = Unbundle By Name(w415) -> ("SCC Ref"=w413:T4, "Paths.Package Spec file path"=w416:path)
        n165 = Build Array(w416) -> (w412:path[])
        n166 = call <vilib>:"SCC Undo Check Out.vi"("error in (no error)"=w411, "files"=w412, "source control reference in"=w413) -> ("error out"=w410:errorcluster, "source control reference out"=w409:T4)  [unwired: 5 in, 2 out]
        n167 = Bundle By Name(cluster=w415, "SCC Ref"=w409) -> (w414:T5)
        n168 = call <vilib>:"Add State(s) to Queue__jki_lib_state_machine.vi"("State(s) in (\"\")"=w418) -> ("States Out"=w417:string)  [unwired: 14 in]
      }
      frame "Project: Set Build Number" {
        n169 = Unbundle By Name(w420) -> ("Proj Item"=w424:refnum<vi>, "CmdLineArgs.BuildNumber"=w428:u32)
        n170 = call "Executable Get Version__icon_lib_labview_project_api.vi"("error in (no error)"=w423, "Build Spec Reference"=w424) -> ("error out"=w425:errorcluster, "Version"=w429:T9, "Build Spec Reference Dup"=w426:refnum<vi>)  [unwired: 7 in]
        n171 = Bundle By Name(cluster=w429, "Build"=w428) -> (w427:T9)
        n172 = call "Executable Set Version__icon_lib_labview_project_api.vi"("error in (no error)"=w425, "Version"=w427, "Build Spec Reference"=w426) -> ("error out"=w422:errorcluster, "Build Spec Reference Dup"=w421:refnum<vi>)  [unwired: 7 in]
        n173 = Bundle By Name(cluster=w420, "Proj Item"=w421) -> (w419:T5)
        n174 = call <vilib>:"Add State(s) to Queue__jki_lib_state_machine.vi"("State(s) in (\"\")"=w431) -> ("States Out"=w430:string)  [unwired: 14 in]
      }
      frame "Project: Enable Logfile" {
        n175 = Unbundle By Name(w438) -> ("Proj Item"=w436:refnum<vi>)
        n176 = call "Executable Set Logfile.vi"("error in (no error)"=w434, "relative Path"=path "build-specs/logfile.txt", "Build Spec Reference"=w436) -> ("error out"=w433:errorcluster, "Build Spec Reference Dup"=w435:refnum<vi>)  [unwired: 7 in]
        n177 = Bundle By Name(cluster=w438, "Proj Item"=w435) -> (w437:T5)
        n178 = call <vilib>:"Add State(s) to Queue__jki_lib_state_machine.vi"("State(s) in (\"\")"=w440) -> ("States Out"=w439:string)  [unwired: 14 in]
      }
      frame "Project: Set Installer Build Dir" {
        n179 = Unbundle By Name(w447) -> ("Proj Item"=w445:refnum<vi>)
        n180 = call "Installer Set Build Directory.vi"("error in (no error)"=w442, "relative Path"=path "installer", "Build Spec Reference"=w445) -> ("error out"=w443:errorcluster, "Build Spec Reference Dup"=w444:refnum<vi>)  [unwired: 7 in]
        n181 = Bundle By Name(cluster=w447, "Proj Item"=w444) -> (w446:T5)
        n182 = call <vilib>:"Add State(s) to Queue__jki_lib_state_machine.vi"("State(s) in (\"\")"=w449) -> ("States Out"=w448:string)  [unwired: 14 in]
      }
      frame "Project: Get Project Item" {
        n183 = Unbundle By Name(w457) -> ("Proj Ref"=w460:refnum<vi>, "Proj Item"=w459:refnum<vi>)
        n184 = Close Reference(reference=w459, error in (no error)=w458) -> (error out=w455:errorcluster)
        n185 = call <vilib>:"Clear Errors.vi"("error in (no error)"=w455) -> ("error out"=w454:errorcluster)  [unwired: 5 in, 1 out]
        n186 = call "Get My Computer Build Spec Children__icon_lib_labview_project_api.vi"("error in (no error)"=w454, "Project Reference"=w460) -> ("error out"=w462:errorcluster, "Children[]"=w463:refnum<vi>[])  [unwired: 7 in, 1 out]
        n187 = for {
          shift-right: [w478] -> w461
          shift-left: w462 -> [w480]
          tunnel: w463 -> [w479] mode=indexing
          tunnel: [w477] -> w466 mode=indexing
          tunnel: [w476] -> w465 mode=indexing
          n188 = property class="ProjectItem"(reference=w479, error in=w480) -> (reference out=w477:refnum<vi>, error out=w478:errorcluster, "Name"=w476:string)
        }
        n189 = Search 1D Array(1D array=w465, element=w468) -> (index of element=w467:i32)  [unwired: 1 out]
        n190 = Delete From Array(array=w466, index=w467) -> (deleted portion=w453:refnum<vi>, array with subset deleted=w464:refnum<vi>[])  [unwired: 1 in]
        n191 = Not A Number/Path/Refnum?(number/path/refnum=w453) -> (NaN/Path/Refnum?=w452:bool)
        n192 = Close Reference(reference=w464, error in (no error)=w461) -> (error out=w451:errorcluster)
        n193 = case shown="True" w452 {
          tunnel: w451 -> [w471 w475]
          tunnel: [w471 w474] -> w450
          frame False {
          }
          frame True {
            w472 = 42 items=["No error", "Argument error", "Memory is full", "Out of zone", "End of file", "File already open", "Generic file I/O error", "File not found", "File permission error", "Disk is full", "Duplicate path", "Too many files open", "System feature not enabled", "Resource file not found", "Cannot add resource", "Resource not found", "Image not found", "Image memory error", "Pen does not exist", "Config type invalid", "Config token not found", "Config parse error", "Config memory error", "Bad external code format", "Bad external code offset", "External code not present", "Null window", "Destroy window error", "Null menu", "Print aborted", "Bad print record", "Print driver error", "Windows error during printing", "Memory error during printing", "Print dialog error", "Generic print error", "Invalid device refnum", "Device not found", "Device parameter error", "Device unit error", "Cannot open device", "Device call aborted", "Generic error", "Cancelled by user", "Object ID too low", "Object ID too high", "Object not in heap", "Unknown heap", "Unknown object (invalid DefProc)", "Unknown object (DefProc not in table)", "Message out of range", "Invalid (null) method", "Unknown message", "Manager call not supported", "Bad address", "Network operation in progress", "Network operation timed out", "Connection is busy", "Network attribute not supported", "Network error", "Address in use", "System out of memory", "Connection aborted", "Connection refused", "Not connected", "Already connected", "Connection closed", "Initialization error (interapplication manager)", "Bad occurrence", "Wait on unbound occurrence handler", "Occurrence queue overflow", "Datalog type conflict", "Unused", "Unrecognized type (interapplication manager)", "Memory corrupt", "Failed to make temporary DLL", "Old CIN version", "Drag socket not found", "Failed to load drop-object", "Failed to register OLE object", "Failed to release OLE object", "Format specifier type mismatch", "Unknown format specifier", "Too few format specifiers", "Too many format specifiers", "Scan failed", "Newer CIN version", "Error converting to variant", "Runtime menu error", "Password tampered", "Variant attribute not found", "Incompatible variant data type", "Event data is not available", "Event Store is not present", "Occurrence is not found", "Event Queue is not created", "Event info is not available", "Refnum passed is NULL", "Error retrieving Class GUID", "Error retrieving CoClass GUID", "Error retrieving TypeLib GUID.", "Bad built application magic bytes.", "Specific driver is different from the specific driver associated with the Logical Name.", "There is no session opened to the class driver.", "Max Error", "MAX - Error with config objects", "MAX - Error loading configuration", "MAX - Group not supported"]
            n194 = call <vilib>:"Error Cluster From Error Code.vi"("error in (no error)"=w475, "error message (\"\")"="Build specification not found in project file" ("error message (\"\")"), "error code (0)"=w472) -> ("error out"=w474:errorcluster)  [unwired: 6 in]
          }
        }
        n195 = Bundle By Name(cluster=w457, "Proj Item"=w453) -> (w456:T5)
        n196 = call <vilib>:"Add State(s) to Queue__jki_lib_state_machine.vi"("State(s) in (\"\")"=w470) -> ("States Out"=w469:string)  [unwired: 14 in]
      }
    }
  }
